vi "Build One Term Compare Abstract Types.vi"   [LabVIEW 2019]
uses:
  <vilib>/Utility/miscctls.llb/LVPointTypeDef.ctl
  <vilib>/numeric/LVNumericRepresentation.ctl
  71b9e51f-dfc8-458f-9837-ddab78837e89.vi
  89ad8fd7-fbe2-448d-841e-7daef20a0f7b.vi
types:
  T1 = typedef "LVNumericRepresentation.ctl" = enum32{"Extended Precision", "Double Precision", "Single Precision", "Long", "Word", "Byte", "Unsigned Long", "Unsigned Word", "Unsigned Byte", "Complex Extended", "Complex Double", "Complex Single", "Quad", "Unsigned Quad", "Fixed-Point"}
  T2 = typedef "LVPointTypeDef.ctl" = cluster{"Horizontal":i16, "Vertical":i16}
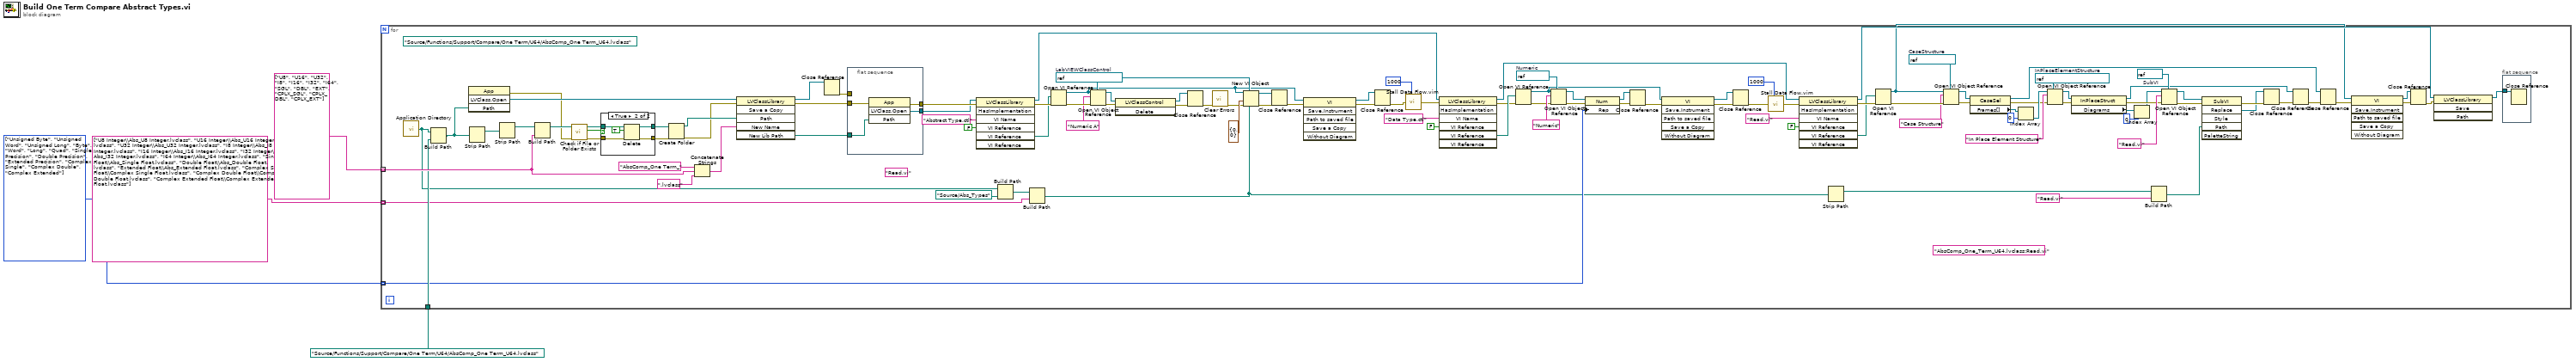
[diagram p0: block diagram]
diagram:
  w1 = T1[] [enum."Unsigned Byte", enum."Unsigned Word", enum."Unsigned Long", enum."Byte", enum."Word", enum."Long", enum."Quad", enum."Single Precision", enum."Double Precision", enum."Extended Precision", enum."Complex Single", enum."Complex Double", enum."Complex Extended"] items=["Extended Precision", "Double Precision", "Single Precision", "Long", "Word", "Byte", "Unsigned Long", "Unsigned Word", "Unsigned Byte", "Complex Extended", "Complex Double", "Complex Single", "Quad", "Unsigned Quad", "Fixed-Point"] ("Representation")
  n1 = for {
    tunnel: string[] ["U8", "U16", "U32", "I8", "I16", "I32", "I64", "SGL", "DBL", "EXT", "CPLX_SGL", "CPLX_DBL", "CPLX_EXT"] -> [w107] mode=indexing
    tunnel: path "Source/Functions/Support/Compare/One Term/U64/AbsComp_One Term_U64.lvclass" -> [w98]
    tunnel: string[] ["U8 Integer\\Abs_U8 Integer.lvclass", "U16 Integer\\Abs_U16 Integer.lvclass", "U32 Integer\\Abs_U32 Integer.lvclass", "I8 Integer\\Abs_I8 Integer.lvclass", "I16 Integer\\Abs_I16 Integer.lvclass", "I32 Integer\\Abs_I32 Integer.lvclass", "I64 Integer\\Abs_I64 Integer.lvclass", "Single Float\\Abs_Single Float.lvclass", "Double Float\\Abs_Double Float.lvclass", "Extended Float\\Abs_Extended Float.lvclass", "Complex Single Float\\Complex Single Float.lvclass", "Complex Double Float\\Complex Double Float.lvclass", "Complex Extended Float\\Complex Extended Float.lvclass"] -> [w88] mode=indexing
    tunnel: w1 -> [w65] mode=indexing
    w36 = refnum<vi> refnum  # InPlaceElementStructure
    w38 = refnum<vi> refnum  # CaseStructure
    (unwired) "AbsComp_One_Term_U64.lvclass:Read.vi" ("name/order")
    w42 = refnum<vi> refnum  # SubVI
    w66 = refnum<vi> refnum  # Numeric
    w80 = refnum<vi> refnum  # LabVIEWClassControl
    (unwired) "Read.vi"
    (unwired) path "Source/Functions/Support/Compare/One Term/U64/AbsComp_One Term_U64.lvclass"
    n2 = call <vilib>:"Application Directory.vi"() -> ("Application Directory"=w91:path)
    n3 = Build Path(base path=w91, name or relative path=w98) -> (appended path=w99:path)
    n4 = invoke class="App" method="LVClass.Open"("Path"=w99) -> (error out=w104:errorcluster, "LVClass.Open"=w118:refnum<vi>)  [unwired: 3 in, 2 out]
    n5 = Strip Path(path=w99) -> (stripped path=w116:path)  [unwired: 1 out]
    n6 = Strip Path(path=w116) -> (stripped path=w115:path)  [unwired: 1 out]
    n7 = Build Path(base path=w115, name or relative path=w107) -> (appended path=w111:path)
    n8 = call <vilib>:"Check if File or Folder Exists.vi"("error in (no error)"=w104, "path"=w111) -> ("error out"=w103:errorcluster, "file or folder exists?"=w113:bool, "dup path"=w114:path)  [unwired: 7 in]
    n9 = case shown="True" w113 {
      tunnel: w114 -> [w125 w130]
      tunnel: [w125 w128] -> w112
      tunnel: w103 -> [w124 w127]
      tunnel: [w124 w126] -> w102
      frame False {
      }
      frame True {
        n10 = Delete(path (use dialog)=w130, entire hierarchy (F)=TRUE, error in=w127) -> (deleted path=w128:path, error out=w126:errorcluster)  [unwired: 2 in, 1 out]
      }
    }
    n11 = Create Folder(path (use dialog)=w112, error in=w102) -> (created path=w110:path, error out=w101:errorcluster)  [unwired: 1 in, 1 out]
    n12 = Concatenate Strings("AbsComp_One Term_", w107, ".lvclass") -> (w97:string)
    n13 = invoke class="LVClassLibrary" method="Save a Copy"(reference=w118, error in=w101, "Path"=w110, "New Name"=w97) -> (reference out=w117:refnum<vi>, error out=w105:errorcluster, "New Lib Path"=w106:path)  [unwired: 2 in, 3 out]
    n14 = Close Reference(reference=w117) -> (error out=w100:errorcluster)  [unwired: 1 in]
    n15 = flat-sequence {
      tunnel: w106 -> [w122]
      tunnel: w105 -> [w123]
      tunnel: w100 -> [_]
      tunnel: [w120] -> w74
      tunnel: [w121] -> w96
      frame #0 {
        n16 = invoke class="App" method="LVClass.Open"(error in=w123, "Path"=w122) -> (error out=w121:errorcluster, "LVClass.Open"=w120:refnum<vi>)  [unwired: 2 in, 2 out]
      }
    }
    n17 = invoke class="LVClassLibrary" method="HasImplementation"(reference=w74, error in=w96, "VI Name"="Abstract Type.ctl", "VI Reference"=FALSE ("Consider Parents?")) -> (reference out=w53:refnum<vi>, error out=w94:errorcluster, "VI Reference"=w93:path)  [unwired: 3 in, 4 out]
    n18 = Build Path(base path=w91, name or relative path=path "Source/Abs_Types") -> (appended path=w89:path)
    n19 = Build Path(base path=w89, name or relative path=w88) -> (appended path=w46:path)
    n20 = Open VI Reference(vi path=w93, error in (no error)=w94) -> (vi reference=w7:refnum<vi>, error out=w87:errorcluster)  [unwired: 4 in]
    n21 = Open VI Object Reference(7:w80, 8:w87, 10:"Numeric A" ("name/order"), 11:w7) -> (0:w85:errorcluster, 3:w84:refnum<vi>)
    n22 = invoke class="LVClassControl" method="Delete"(reference=w84, error in=w85) -> (reference out=w83:refnum<vi>, error out=w78:errorcluster)  [unwired: 1 in, 1 out]
    n23 = Close Reference(reference=w83, error in (no error)=w78) -> (error out=w77:errorcluster)
    n24 = call <vilib>:"Clear Errors.vi"("error in (no error)"=w77) -> ("error out"=w76:errorcluster)  [unwired: 5 in, 1 out]
    n25 = New VI Object(vi object class=w80, owner refnum=w7, position/next to=T2 {"Horizontal"=0, "Vertical"=0} ("location"), 6:w46, 8:w76) -> (object refnum=w81:refnum<vi>, 0:w82:errorcluster)  [unwired: 3 in]
    n26 = Close Reference(reference=w81, error in (no error)=w82) -> (error out=w8:errorcluster)
    n27 = invoke class="VI" method="Save.Instrument"(reference=w7, error in=w8) -> (reference out=w5:refnum<vi>, error out=w6:errorcluster)  [unwired: 4 in, 4 out]
    n28 = Close Reference(reference=w5, error in (no error)=w6) -> (error out=w62:errorcluster)
    n29 = call "Stall Data Flow.vim"("value in"=w62, "milliseconds to wait"=u32 1000) -> ("value out"=w61:errorcluster)  [unwired: 1 out]
    n30 = invoke class="LVClassLibrary" method="HasImplementation"(reference=w53, error in=w61, "VI Name"="Data Type.ctl", "VI Reference"=FALSE ("Consider Parents?")) -> (reference out=w54:refnum<vi>, error out=w71:errorcluster, "VI Reference"=w72:path)  [unwired: 3 in, 4 out]
    n31 = Open VI Reference(vi path=w72, error in (no error)=w71) -> (vi reference=w11:refnum<vi>, error out=w69:errorcluster)  [unwired: 4 in]
    n32 = Open VI Object Reference(7:w66, 8:w69, 10:"Numeric" ("name/order"), 11:w11) -> (0:w68:errorcluster, 3:w67:refnum<vi>)
    n33 = property class="Num"(reference=w67, error in=w68, "Rep"=w65) -> (reference out=w63:refnum<vi>, error out=w64:errorcluster)
    n34 = Close Reference(reference=w63, error in (no error)=w64) -> (error out=w12:errorcluster)
    n35 = invoke class="VI" method="Save.Instrument"(reference=w11, error in=w12) -> (reference out=w10:refnum<vi>, error out=w9:errorcluster)  [unwired: 4 in, 4 out]
    n36 = Close Reference(reference=w10, error in (no error)=w9) -> (error out=w58:errorcluster)
    n37 = call "Stall Data Flow.vim"("value in"=w58, "milliseconds to wait"=u32 1000) -> ("value out"=w56:errorcluster)  [unwired: 1 out]
    n38 = invoke class="LVClassLibrary" method="HasImplementation"(reference=w54, error in=w56, "VI Name"="Read.vi", "VI Reference"=FALSE ("Consider Parents?")) -> (reference out=w21:refnum<vi>, error out=w52:errorcluster, "VI Reference"=w51:path)  [unwired: 3 in, 4 out]
    n39 = Strip Path(path=w46) -> (stripped path=w45:path)  [unwired: 1 out]
    n40 = Open VI Reference(vi path=w51, error in (no error)=w52) -> (vi reference=w18:refnum<vi>, error out=w41:errorcluster)  [unwired: 4 in]
    n41 = Open VI Object Reference(7:w38, 8:w41, 10:"Case Structure" ("name/order"), 11:w18) -> (0:w35:errorcluster, 3:w34:refnum<vi>)
    n42 = property class="CaseSel"(reference=w34, error in=w35) -> (reference out=w19:refnum<vi>, error out=w30:errorcluster, "Frames[]"=w33:refnum<vi>[])
    n43 = Index Array(array=w33, index=0) -> (element=w31:refnum<vi>)
    n44 = Open VI Object Reference(7:w36, 8:w30, 10:"In Place Element Structure" ("name/order"), 11:w31) -> (0:w28:errorcluster, 3:w27:refnum<vi>)
    n45 = property class="InPlaceStruct"(reference=w27, error in=w28) -> (reference out=w22:refnum<vi>, error out=w24:errorcluster, "Diagrams"=w26:refnum<vi>[])
    n46 = Index Array(array=w26, index=0) -> (element=w23:refnum<vi>)
    n47 = Build Path(base path=w45, name or relative path="Read.vi") -> (appended path=w43:path)
    n48 = Open VI Object Reference(7:w42, 8:w24, 10:"Read.vi" ("name/order"), 11:w23) -> (0:w37:errorcluster, 3:w50:refnum<vi>)
    n49 = invoke class="SubVI" method="Replace"(reference=w50, error in=w37, "Path"=w43) -> (error out=w49:errorcluster, "Replace"=w48:refnum<vi>)  [unwired: 3 in, 4 out]
    n50 = Close Reference(reference=w48, error in (no error)=w49) -> (error out=w47:errorcluster)
    n51 = Close Reference(reference=w22, error in (no error)=w47) -> (error out=w17:errorcluster)
    n52 = Close Reference(reference=w19, error in (no error)=w17) -> (error out=w16:errorcluster)
    n53 = invoke class="VI" method="Save.Instrument"(reference=w18, error in=w16) -> (reference out=w14:refnum<vi>, error out=w15:errorcluster)  [unwired: 4 in, 4 out]
    n54 = Close Reference(reference=w14, error in (no error)=w15) -> (error out=w13:errorcluster)
    n55 = invoke class="LVClassLibrary" method="Save"(reference=w21, error in=w13) -> (reference out=w20:refnum<vi>)  [unwired: 2 in, 3 out]
    n56 = flat-sequence {
      tunnel: w20 -> [w119]
      frame #0 {
        n57 = Close Reference(reference=w119) -> ()  [unwired: 1 in, 1 out]
      }
    }
  }
